vi "initHandler.vi"(8 "error in (no error)":errorcluster, 9 "Name":string, 10 "Level":T1(ring), 11 "Handler.File in":refnum<class "Handler.File.lvclass">) -> (0 "error out":errorcluster, 3 "Handler.File out":refnum<class "Handler.File.lvclass">)   [LabVIEW 2017, in "Error Log.lvlib" / "Handler.File.lvclass"]
uses:
  Handler.File.lvclass
  Handler/Handler.lvclass
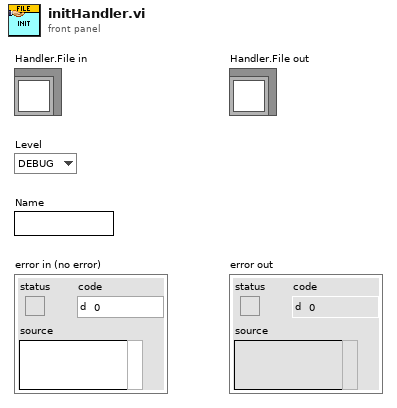
[diagram p1: front panel]
types:
  T1 = enum16{"DEBUG", "INFO", "WARNING", "ERROR", "CRITICAL"}
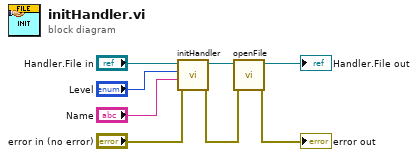
[diagram p0: block diagram]
diagram:
  n1 = call-parent "initHandler.vi"("error in (no error)"="error in (no error)", "Name"="Name", "Level"="Level", "Handler in"="Handler.File in") -> ("error out"=w3:errorcluster, "Handler out"=w4:refnum<class "Handler.File.lvclass">)  [unwired: 6 in]
  n2 = call-dynamic "openFile.vi"("error in (no error)"=w3, "Handler.File in"=w4) -> ("error out"=→"error out":errorcluster, "Handler.File out"=→"Handler.File out":refnum<class "Handler.File.lvclass">)  [unwired: 8 in]
